vi "FGV-MassData.vi"(6 "Operation":T1, 8 "Error in":errorcluster caption="Error in (no error)", 9 "size":i32, 10 "Start":i32, 11 "Data in":dbl[](array[numeric])) -> (0 "Error out":errorcluster, 1 "Active Read Oper":T2, 2 "Active Write Oper":T2, 3 "Data out":dbl[](array[numeric]) format="%.2f", 4 "Cache Size":i32)   [LabVIEW 2014, in "JKISM++ Array Parameter Support.lvlib"]
uses:
  JKISM++ Array Parameter Support.lvlib
  Def-MassDataOper-Status.ctl
  Operation-FGV-MassData.ctl
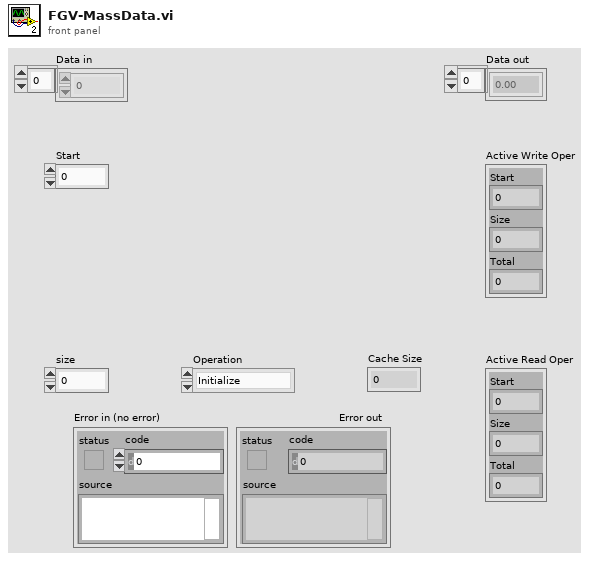
[diagram p1: front panel]
types:
  T1 = typedef "JKISM++ Array Parameter Support.lvlib/Operation-FGV-MassData.ctl" = enum16{"Initialize", "Read", "Write", "Status", "Release"}
  T2 = typedef "JKISM++ Array Parameter Support.lvlib/Def-MassDataOper-Status.ctl" = cluster{"Start":i32, "Size":i32, "Total":i32}
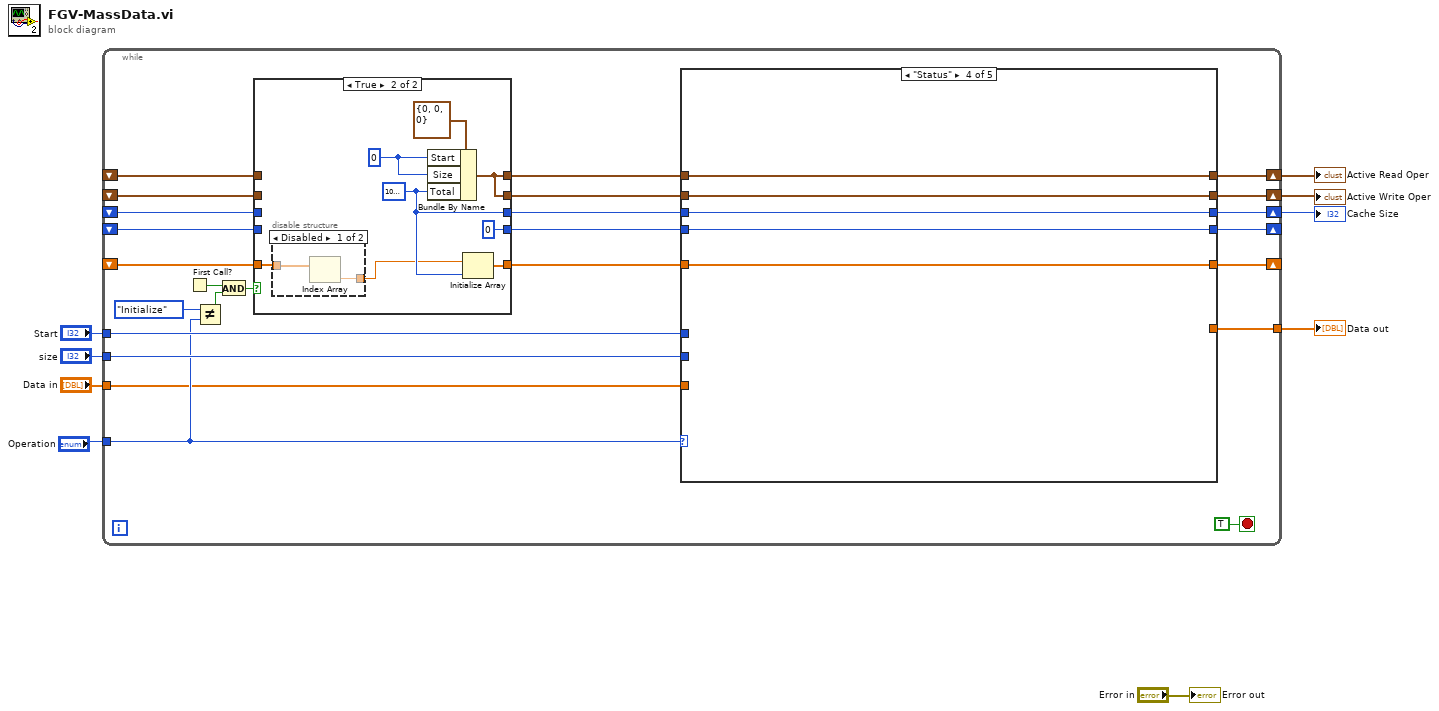
[diagram p0: block diagram]
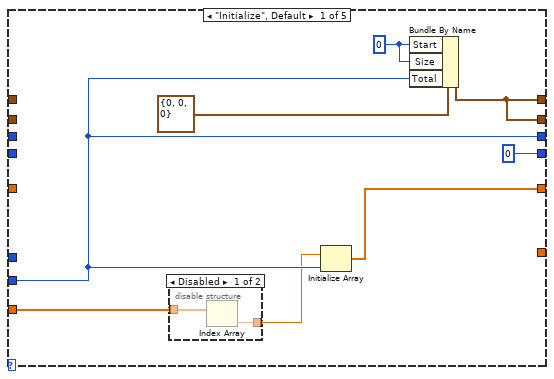
[diagram p4: hidden frame]
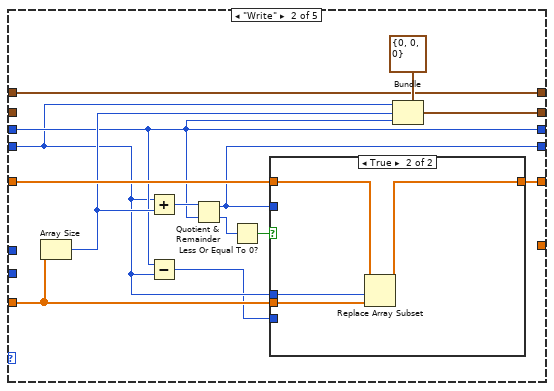
[diagram p6: hidden frame]
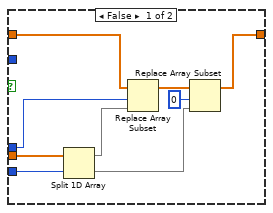
[diagram p7: hidden frame]
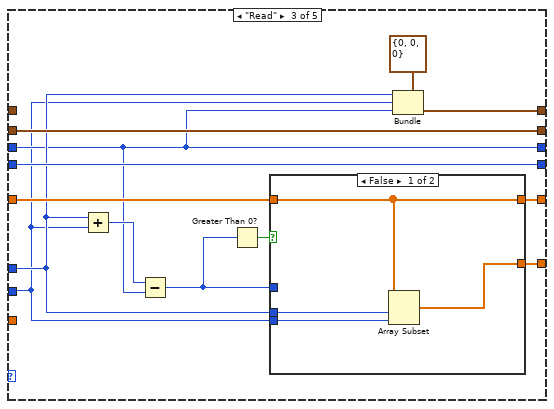
[diagram p8: hidden frame]
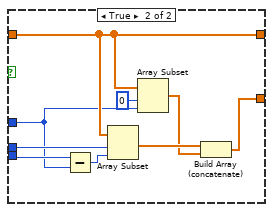
[diagram p9: hidden frame]
diagram:
  n1 = while {
    tunnel: "Operation" -> [w23]
    shift-right: [w33] -> _
    shift-left: _ -> [w11]
    tunnel: "Start" -> [w32]
    tunnel: "size" -> [w31]
    tunnel: [w30] -> w6
    tunnel: "Data in" -> [w10]
    shift-right: [w29] -> w1
    shift-left: _ -> [w14]
    shift-right: [w28] -> w3
    shift-left: _ -> [w17]
    shift-right: [w27] -> w4
    shift-left: _ -> [w20]
    shift-right: [w26] -> _
    shift-left: _ -> [w13]
    stop <- TRUE stop-if-true
    n2 = First Call?() -> (First Call?: T/F=w25:bool)
    n3 = Not Equal?(x=Operation-FGV-MassData."Initialize", y=w23) -> (x != y?=w24:bool)
    n4 = And(x=w25, y=w24) -> (x .and. y?=w21:bool)
    n5 = case shown="True" w21 {
      tunnel: w20 -> [w39 _]
      tunnel: [w39 w43] -> w19
      tunnel: [w38 w43] -> w18
      tunnel: w17 -> [w38 _]
      tunnel: [w37 w44] -> w16
      tunnel: [w36 0 ("Start")] -> w15
      tunnel: w14 -> [w37 _]
      tunnel: w13 -> [w36 _]
      tunnel: [w35 w47] -> w12
      tunnel: w11 -> [w35 w41]
      frame False {
      }
      frame True {
        w45 = 0 ("Start")
        w44 = 1000000
        n6 = disable-structure shown="Disabled" {
          disable-tunnel: w41 -> [w49 _]
          disable-tunnel: [w48 _] -> w40
          frame Disabled {
            n7 = Index Array(array=w49) -> (element=w48:dbl)  [unwired: 1 in]
          }
          frame Enabled {
          }
        }
        n8 = Bundle By Name(cluster=T2 {"Start"=0, "Size"=0, "Total"=0} ("Cache Status"), "Start"=w45, "Size"=w45, "Total"=w44) -> (w43:T2)
        n9 = Initialize Array(w40, w44) -> (w47:dbl[])
      }
    }
    n10 = case shown="\"Status\"" w23 {
      tunnel: [w54 w72 w98 w117 w122] -> w33
      tunnel: w12 -> [_ w73 w99 w117 w122]
      tunnel: w32 -> [_ _ w92 _ _]
      tunnel: w31 -> [w55 _ w88 _ _]
      tunnel: [_ _ w87 _ _] -> w30
      tunnel: w10 -> [w51 w71 _ _ _]
      tunnel: [w55 w62 w90 w113 w121] -> w29
      tunnel: w16 -> [_ w62 w90 w113 w121]
      tunnel: [w56 w69 w94 w116 w120] -> w28
      tunnel: w18 -> [_ _ w94 w116 w120]
      tunnel: [w56 w68 w95 w115 w119] -> w27
      tunnel: w19 -> [_ w68 _ w115 w119]
      tunnel: w15 -> [_ w61 w93 w114 w118]
      tunnel: [0 ("Start") w64 w93 w114 w118] -> w26
      frame "Initialize", Default {
        w57 = 0 ("Start")
        n11 = disable-structure shown="Disabled" {
          disable-tunnel: w51 -> [w59 _]
          disable-tunnel: [w58 _] -> w50
          frame Disabled {
            n12 = Index Array(array=w59) -> (element=w58:dbl)  [unwired: 1 in]
          }
          frame Enabled {
          }
        }
        n13 = Initialize Array(w50, w55) -> (w54:dbl[])
        n14 = Bundle By Name(cluster=T2 {"Start"=0, "Size"=0, "Total"=0} ("Cache Status"), "Start"=w57, "Size"=w57, "Total"=w55) -> (w56:T2)
      }
      frame "Write" {
        n15 = Array Size(array=w71) -> (size(s)=w63:i32)
        n16 = Add(x=w61, y=w63) -> (x+y=w67:i32)
        n17 = Subtract(x=w62, y=w61) -> (x-y=w60:i32)
        n18 = Quotient & Remainder(x=w67, y=w62) -> (x-y*floor(x/y)=w64:i32, floor(x/y)=w66:i32)
        n19 = Less Or Equal To 0?(x=w66) -> (x <= 0?=w65:bool)
        n20 = case shown="True" w65 {
          tunnel: w73 -> [w82 w86]
          tunnel: [w78 w85] -> w72
          tunnel: w71 -> [w80 w84]
          tunnel: w61 -> [w81 w83]
          tunnel: w64 -> [_ _]
          tunnel: w60 -> [w74 _]
          frame False {
            n21 = Split 1D Array(array=w80, index=w74) -> (first subarray=w75:dbl[], second subarray=w76:dbl[])
            n22 = Replace Array Subset(array=w82, new element=w75, index=w81) -> (w79:dbl[])
            n23 = Replace Array Subset(array=w79, new element=w76, index=0) -> (w78:dbl[])
          }
          frame True {
            n24 = Replace Array Subset(array=w86, new element=w84, index=w83) -> (w85:dbl[])
          }
        }
        n25 = Bundle(cluster=T2 {"Start"=0, "Size"=0, "Total"=0} ("Cache Status"), "Start"=w61, "Size"=w63, "Total"=w62) -> (w69:T2)
      }
      frame "Read" {
        n26 = Add(x=w92, y=w88) -> (x+y=w91:i32)
        n27 = Subtract(x=w91, y=w90) -> (x-y=w89:i32)
        n28 = Greater Than 0?(x=w89) -> (x > 0?=w96:bool)
        n29 = case shown="False" w96 {
          tunnel: w99 -> [w102 w112]
          tunnel: [w102 w112] -> w98
          tunnel: w92 -> [w103 w111]
          tunnel: w89 -> [_ w105]
          tunnel: w88 -> [w101 w106]
          tunnel: [w100 w107] -> w87
          frame False {
            n30 = Array Subset(array=w102, index=w103, length=w101) -> (w100:dbl[])
          }
          frame True {
            n31 = Subtract(x=w106, y=w105) -> (x-y=w104:i32)
            n32 = Array Subset(array=w112, index=w111, length=w104) -> (w109:dbl[])
            n33 = Array Subset(array=w112, index=0, length=w105) -> (w108:dbl[])
            n34 = Build Array (concatenate)(w109, w108) -> (w107:dbl[])
          }
        }
        n35 = Bundle(cluster=T2 {"Start"=0, "Size"=0, "Total"=0} ("Cache Status"), "Start"=w92, "Size"=w88, "Total"=w90) -> (w95:T2)
      }
      frame "Status" {
      }
      frame "Release" {
      }
    }
  }
  "Data out" <- w6
  "Active Read Oper" <- w4
  "Active Write Oper" <- w3
  "Cache Size" <- w1
  "Error out" <- "Error in"
